vi "Flang Controller.vi"(8 "error in":errorcluster) -> ()   [LabVIEW 2019]
doc: "This VI executes continuously carrying out the current operation and responding to updates or new operations. It will often contain the timing or control code that is difficult to place directly in TeleOp. This VI generally opens all sensors and motors and isolates the rest of the robot code from knowing how the operations are carried out."
uses:
  <vilib>/Rock Robotics/WPI/Framework/Completion Status.ctl
  Flang Setpoints.ctl
  Flang Operations.ctl
  <vilib>/Rock Robotics/WPI/ThirdParty/Phoenix-LabVIEW/Motor Controller/Controls/CTRE_Phoenix_MotorControl_ControlMode.ctl
  <vilib>/Rock Robotics/WPI/ThirdParty/Phoenix-LabVIEW/Motor Controller/Get/CTRE_Phoenix_MotorController_GetVoltage.vi
  <vilib>/Rock Robotics/WPI/ThirdParty/Phoenix-LabVIEW/Motor Controller/Get/CTRE_Phoenix_MotorController_GetSelectedSensorData.vi
  <vilib>/Rock Robotics/WPI/ThirdParty/Phoenix-LabVIEW/Motor Controller/Get/CTRE_Phoenix_MotorController_GetSupplyAndStatorCurrent_Enhanced.vi
  <vilib>/Rock Robotics/Network Tables/NT Write Boolean.vi
panel:
  out "Voltage":dbl(graph)
  in  "Setpoint":dbl=0.5
  in  "percent err":dbl=50.0
  out "Position (Raw Sensor Units)":i32
  in  "pid cluster":cluster{"p":dbl, "i":dbl, "d":dbl}
  out "ball in flang":bool
  in  "Expected":dbl=5.7
  out "Pid something":T1(graph)
  out "Supply Current":dbl(graph)
  in  "Interactive Values":T2
  out "Current\nCmd":string
  in  "Buttons":cluster{"Execute Cmd":bool, "Abort Cmd":bool}
  out "Command Timing":cluster{"Start Time (ms)":u32, "Iterations":i32}
  out "Status":T4
  # "Tip: It may be helpful to observe inputs and sensor values.\nYou may also want to display tuning or debugging controls."
  # "Interactive Command: You may fill in the settings for a command\nand schedule it with the Execute button. You can observe and abort\nany command while fine tuning the code for the controller."
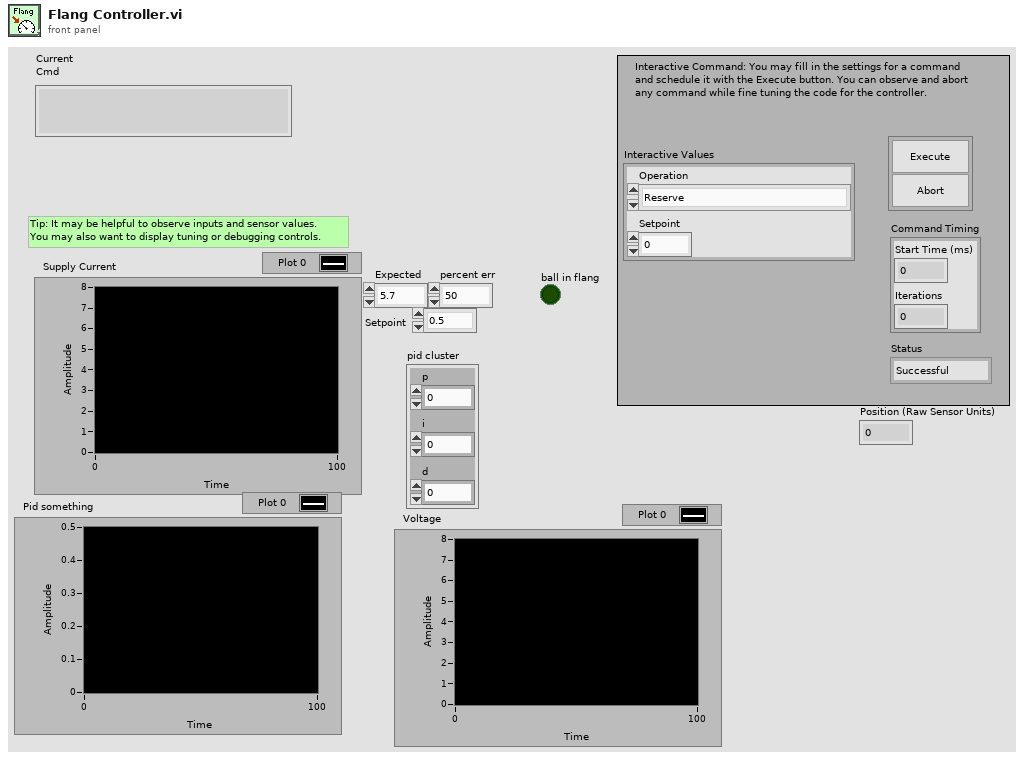
[diagram p1: front panel]
types:
  T1 = cluster{"Setpoint":dbl, "Velocity (Raw Sensor Units per 100 ms)":i32}
  T2 = typedef "Flang Setpoints.ctl" = cluster{"Operation":T3, "Setpoint":dbl}
  T3 = typedef "Flang Operations.ctl" = enum16{"Reserve", "Read Current", "Immediate"}
  T4 = typedef "Completion Status.ctl" = enum16{"Successful", "Aborted", "Incomplete"}
  T5 = typedef "WPI_MotorControlDeviceRef.ctl" = cluster{"DeviceStatus":errorcluster, "Type":T6, "PWM":cluster{"PWM Channel":T7, "DeadBand":T8}, "CAN":cluster{"Device Number":u8, "SetOutput VI Ref":variant, "GetOutput VI Ref":variant, "Enable VI Ref":variant, "Disable VI Ref":variant, "Data":variant}, "Invert":bool, "DIO PWM":cluster{"PWM \"Enable\" Channel":T7, "DIOChannel":T9, "PWM Rate":dbl}}
  T6 = typedef "WPI_MotorControlType.ctl" = enum16{"PWM", "CAN", "DIO PWM"}
  T7 = typedef "FPGA_DIOPWMChannel.ctl" = enum8{"PWM 0", "PWM 1", "PWM 2", "PWM 3", "PWM 4", "PWM 5", "PWM 6", "PWM 7", "PWM 8", "PWM 9", "PWM MXP 0", "PWM MXP 1", "PWM MXP 2", "PWM MXP 3", "PWM MXP 4", "PWM MXP 5", "PWM MXP 6", "PWM MXP 7", "PWM MXP 8", "PWM MXP 9", "Invalid"}
  T8 = typedef "WPI_PWMDeadband.ctl" = cluster{"Name":string, "maxPositivePwm":i32, "minPositivePwm":i32, "centerPwm":i32, "maxNegativePwm":i32, "minNegativePwm":i32, "angularRange":u16}
  T9 = typedef "FPGA_DIOChannel.ctl" = enum8{"DIO 0", "DIO 1", "DIO 2", "DIO 3", "DIO 4", "DIO 5", "DIO 6", "DIO 7", "DIO 8", "DIO 9", "DIO MXP 0", "DIO MXP 1", "DIO MXP 2", "DIO MXP 3", "DIO MXP 4", "DIO MXP 5", "DIO MXP 6", "DIO MXP 7", "DIO MXP 8", "DIO MXP 9", "DIO MXP 10", "DIO MXP 11", "DIO MXP 12", "DIO MXP 13", "DIO MXP 14", "DIO MXP 15", "SPI Port CS1", "SPI Port CS2", "SPI Port CS3", "SPI Port MISO", "SPI Port MOSI", "Invalid"}
  T10 = typedef "Command Status Info.ctl" = cluster{"Name":string, "Status":T4, "notifier out":T11}
  T11 = typedef "Completion Notifier.ctl" = refnum<notifier>
  T12 = cluster{"Current Command":T2, "Command Timing":cluster{"Start Time (ms)":u32, "Iterations":i32}, "Command Arguments":cluster{"Command Info":T10, "Description":string, "Default Command":T2, "queue out":refnum<queue>, "Subsystem Name":string}}
  T13 = typedef "CTRE_Phoenix_MotorControl_ControlMode.ctl" = u16
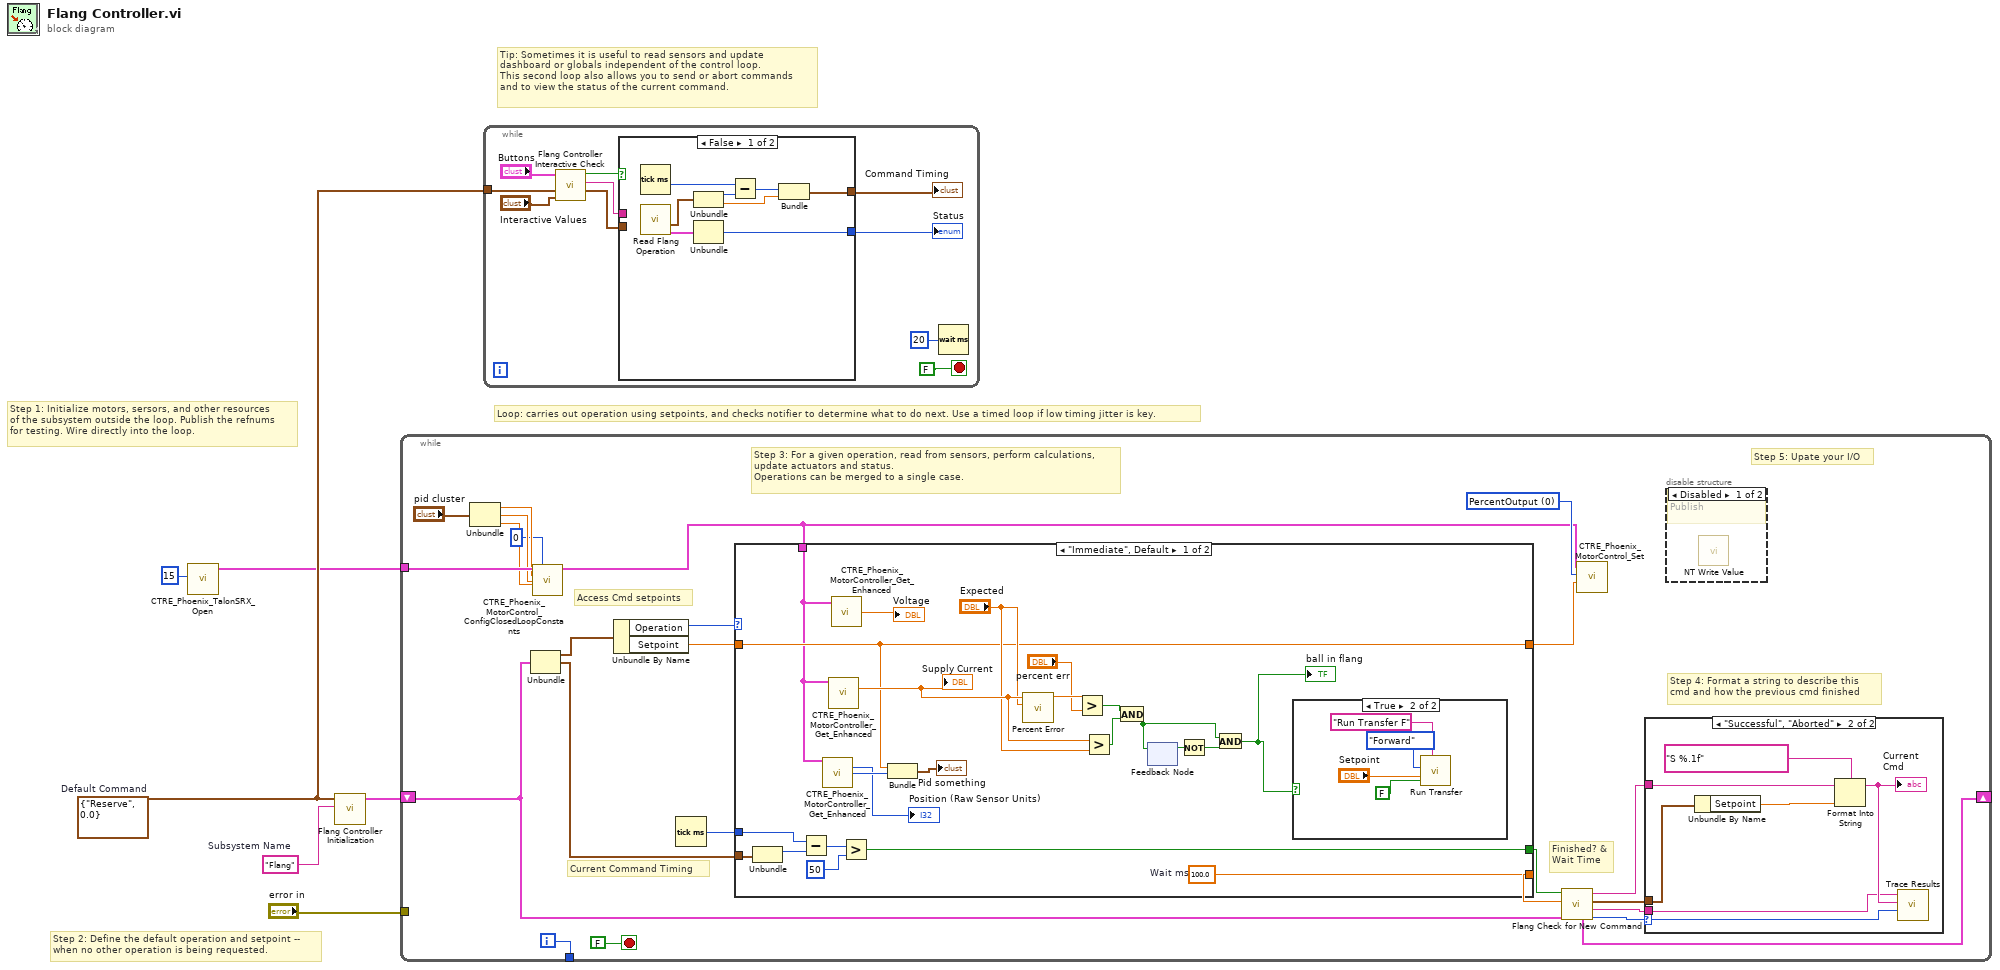
[diagram p0: block diagram]
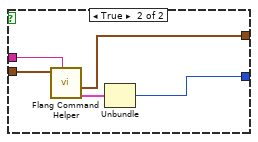
[diagram p2: hidden frame]
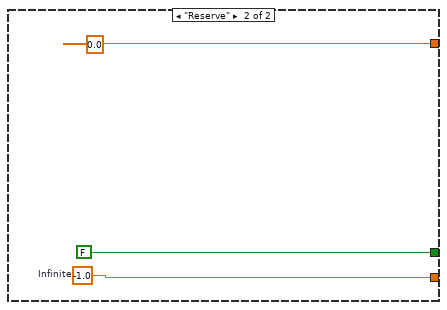
[diagram p6: hidden frame]
diagram:
  w3 = T2 {"Operation"=enum."Reserve", "Setpoint"=0.0}  # Default Command
  w4 = "Flang"  # Subsystem Name
  # "Tip: Sometimes it is useful to read sensors and update\ndashboard or globals independent of the control loop.\nThis second loop also allows you to send or abort commands\nand to view the status of the current command."
  # "Step 2: Define the default operation and setpoint --\nwhen no other operation is being requested."
  # "Step 1: Initialize motors, sersors, and other resources\nof the subsystem outside the loop. Publish the refnums\nfor testing. Wire directly into the loop."
  # "Loop: carries out operation using setpoints, and checks notifier to determine what to do next. Use a timed loop if low timing jitter is key."
  n1 = call <vilib>:"CTRE_Phoenix_TalonSRX_Open.vi"("Device Number"=u8 15) -> ("CAN Talon SRX Ref"=w1:T5)  [unwired: 9 in, 1 out]
  n2 = call "Flang Controller Initialization.vi"("Subsystem Name"=w4, "Default Command"=w3) -> ("Current Command"=w5:T12)  [unwired: 9 in]
  n3 = while {
    shift-right: [w23] -> _
    shift-left: w5 -> [w16]
    tunnel: [w29] -> _
    tunnel: "error in" -> [_]
    tunnel: w1 -> [w13]
    i -> [w29]
    stop <- FALSE stop-if-true
    w14 = T13 0 items=["PercentOutput"=0, "Position"=1, "Velocity"=2, "Current"=3, "Follower"=5, "MotionProfile"=6, "MotionMagic"=7, "MotionProfileArc"=10, "Disabled"=15] ("Control Mode")
    # "Step 5: Upate your I/O"
    # "Step 4: Format a string to describe this\ncmd and how the previous cmd finished"
    # "Current Command Timing"
    # "Access Cmd setpoints"
    # "Finished? &\nWait Time"
    # "Step 3: For a given operation, read from sensors, perform calculations,\nupdate actuators and status.\nOperations can be merged to a single case."
    n4 = Unbundle("pid cluster") -> ("p"=w10:dbl, "i"=w9:dbl, "d"=w8:dbl)
    n5 = Unbundle(w16) -> ("Current Command"=w28:T2, "Command Timing"=w25:cluster{"Start Time (ms)":u32, "Iterations":i32})  [unwired: 1 out]
    n6 = call <vilib>:"CTRE_Phoenix_MotorControl_ConfigClosedLoopConstants.vi"("PhoenixMotorControlDevRef"=w13, "slotIdx"=0, "P"=w10, "I"=w9, "D"=w8) -> ("PhoenixMotorControlDevRef"=w12:T5)  [unwired: 9 in, 1 out]
    n7 = Unbundle By Name(w28) -> ("Operation"=w27:T3, "Setpoint"=w24:dbl)
    n8 = Tick Count (ms)() -> (millisecond timer value=w26:u32)
    n9 = case shown="\"Immediate\", Default" w27 {
      tunnel: [w60 w67] -> w21
      tunnel: [w54 FALSE ("ignore previous (F)")] -> w22
      tunnel: w25 -> [w56 _]
      tunnel: w26 -> [w55 _]
      tunnel: w24 -> [w47 _]
      tunnel: [w47 0.0 ("Setpoint")] -> w15
      tunnel: w12 -> [w39 _]
      frame "Immediate", Default {
        w60 = 100.0  # Wait ms
        n10 = Unbundle(w56) -> ("Start Time (ms)"=w59:u32)  [unwired: 1 out]
        n11 = Subtract(x=w55, y=w59) -> (x-y=w58:u32)
        n12 = call-poly <vilib>:"CTRE_Phoenix_MotorController_Get_Enhanced.vi"("PhoenixMotorControlDevRef"=w39) -> ("Position (Raw Sensor Units)"=→"Position (Raw Sensor Units)":i32, "Velocity (Raw Sensor Units per 100 ms)"=w48:i32)  [unwired: 11 in, 2 out]
        n13 = call-poly <vilib>:"CTRE_Phoenix_MotorController_Get_Enhanced.vi"("PhoenixMotorControlDevRef"=w39) -> ("Supply Current"=w50:dbl)  [unwired: 11 in, 3 out]
        "Supply Current" <- w50
        n14 = call-poly <vilib>:"CTRE_Phoenix_MotorController_Get_Enhanced.vi"("PhoenixMotorControlDevRef"=w39) -> ("Output Voltage"=→"Voltage":dbl)  [unwired: 10 in, 4 out]
        n15 = Greater?(x=w58, y=u8 50 ("Left Motor")) -> (0:w54:bool)
        n16 = Bundle("Setpoint"=w47, "Velocity (Raw Sensor Units per 100 ms)"=w48) -> (→"Pid something":T1)  [unwired: 1 in]
        n17 = call "Percent Error.vi"("Expected"="Expected", "Observed"=w50) -> ("Percent Error"=w53:dbl)  [unwired: 9 in]
        n18 = Greater?(x=w53, y="percent err") -> (0:w52:bool)
        n19 = Greater?(x=w50, y="Expected") -> (0:w51:bool)
        n20 = And(x=w52, y=w51) -> (x .and. y?=w41:bool)
        n21 = feedback-in #1(w41) -> ()
        n22 = feedback #1() -> (w43:bool)  [unwired: 1 in]
        n23 = Not(x=w43) -> (.not. x?=w42:bool)
        n24 = And(x=w41, y=w42) -> (x .and. y?=w40:bool)
        "ball in flang" <- w40
        n25 = case shown="True" w40 {
          frame False {
          }
          frame True {
            n26 = call "Run Transfer.vi"("Description"="Run Transfer F", "Finish?"=FALSE, "Direction"=enum16{"Forward", "Backward"}."Forward", "Setpoint"="Setpoint") -> ()  [unwired: 7 in, 1 out]
          }
        }
      }
      frame "Reserve" {
        w67 = -1.0  # Infinite
      }
    }
    n27 = call "Flang Check for New Command.vi"("Current Command"=w16, "Wait time (ms)"=w21, "Finished?"=w22) -> ("Completion"=w17:T4, "Subsystem Name"=w18:string, "Current Command"=w19:T2, "Initial Trace String"=w20:string, "NextCommand"=w23:T12)  [unwired: 4 in]
    n28 = call <vilib>:"CTRE_Phoenix_MotorControl_Set.vi"("Output"=w15, "Control Mode"=w14, "PhoenixMotorControlDevRef"=w12) -> ()  [unwired: 7 in, 2 out]
    n29 = case shown="\"Successful\", \"Aborted\"" w17 {
      selector: w17 -> [_ w37]
      tunnel: w20 -> [_ w33]
      tunnel: w19 -> [_ w34]
      tunnel: w18 -> [_ w31]
      frame "Incomplete", Default {
        # "Continuing current command"
      }
      frame "Successful", "Aborted" {
        # "Report and setup for next command"
        n30 = Unbundle By Name(w34) -> ("Setpoint"=w36:dbl)
        n31 = Format Into String(format string="S %.1f", initial string=w33, w36) -> (resulting string=w32:string)  [unwired: 1 in, 1 out]
        "Current\nCmd" <- w32
        n32 = call <vilib>:"Trace Results.vi"("Status of previous command"=w37, "Description"=w32, "Subsystem"=w31) -> ()  [unwired: 9 in]
      }
    }
    n33 = disable-structure shown="Disabled" {
      frame Disabled {
        # "Publish"
        n34 = call-poly <vilib>:"NT Write Value.vi"() -> ()  [unwired: 11 in, 1 out]
      }
      frame Enabled {
      }
    }
  }
  n35 = while {
    tunnel: w3 -> [w74]
    stop <- FALSE stop-if-true
    n36 = call "Flang Controller Interactive Check.vi"("Interactive Command in"="Interactive Values", "Default Command"=w74, "Buttons"="Buttons") -> ("Interactive Command out"=w71:T2, "Trace String"=w72:string, "Schedule"=w73:bool)  [unwired: 6 in]
    n37 = case shown="False" w73 {
      tunnel: [w85 w90] -> w70
      tunnel: w71 -> [_ w88]
      tunnel: [w81 w86] -> w69
      tunnel: w72 -> [_ w89]
      frame False {
        n38 = Tick Count (ms)() -> (millisecond timer value=w80:u32)
        n39 = call "Read Flang Operation.vi"() -> ("Command Info"=w78:T10, "SubSystem Data"=w79:T2)  [unwired: 9 in, 1 out]
        n40 = Unbundle(w79) -> ("Operation"=w84:T3, "Setpoint"=w82:dbl)
        n41 = Unbundle(w78) -> ("Status"=w85:T4)  [unwired: 2 out]
        n42 = Subtract(x=w80, y=w84) -> (x-y=w83:u32)
        n43 = Bundle(w83, "Setpoint"=w82) -> (w81:cluster{u32, "Setpoint":dbl})  [unwired: 1 in]
      }
      frame True {
        n44 = call "Flang Command Helper.vi"("Description"=w89, "SubSystem Data"=w88) -> ("Command Info Out"=w87:T10, "Command Timing"=w86:cluster{"Start Time (ms)":u32, "Iterations":i32})  [unwired: 7 in, 1 out]
        n45 = Unbundle(w87) -> ("Status"=w90:T4)  [unwired: 2 out]
      }
    }
    "Status" <- w70
    "Command Timing" <- w69
    n46 = Wait (ms)(milliseconds to wait=u32 20) -> ()  [unwired: 1 out]
  }
